vi "RSZVB Set PI Controller Mode.vi"(7 "PI Controller Mode (Auto)":i32(ring) items=["Auto", "Manual"], 8 "error in (no error)":errorcluster {"code" format="%.0x"}, 9 "Port (1)":i32=1, 10 "Channel (1)":i32=1, 11 "VISA session":refnum<visa-resource-name>) -> (0 "error out":errorcluster {"code" format="%.0x"}, 3 "dup VISA session":refnum<visa-resource-name>)   [LabVIEW 2011]
doc: "Enables automatic or manual setting of the PI controller parameters at source port <Pt>. \n\nRemote-control command(s):\nSOURce<Ch>:POWer<Pt>:ALC:PIParameter"
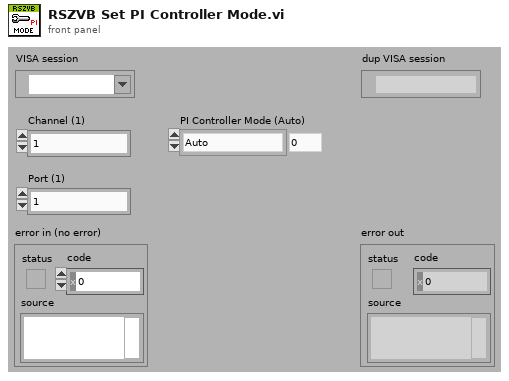
[diagram p1: front panel]
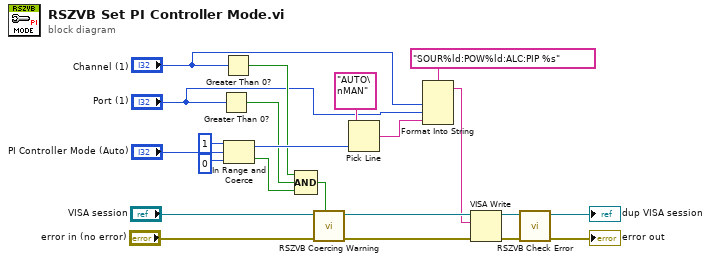
[diagram p0: block diagram]
diagram:
  n1 = Greater Than 0?(x="Port (1)") -> (x > 0?=w9:bool)
  n2 = Greater Than 0?(x="Channel (1)") -> (x > 0?=w10:bool)
  n3 = In Range and Coerce(upper limit=1, x="PI Controller Mode (Auto)", lower limit=0) -> (coerced(x)=w19:i32, In Range?=w8:bool)
  n4 = Compound Arithmetic op=AND(w10, w9, w8) -> (w7:bool)
  n5 = call "RSZVB Coercing Warning.vi"("In Range?"=w7, "error in (no error)"="error in (no error)", "VISA session"="VISA session") -> ("error out"=w16:errorcluster, "dup VISA session"=w17:refnum<visa-resource-name>)  [unwired: 7 in]
  n6 = Pick Line(multi-line string="AUTO\nMAN", line index=w19) -> (output string=w11:string)  [unwired: 1 in]
  n7 = Format Into String(format string="SOUR%ld:POW%ld:ALC:PIP %s", "Channel (1)", "Port (1)", w11) -> (resulting string=w13:string)  [unwired: 2 in, 1 out]
  n8 = VISA Write(VISA resource name=w17, write buffer=w13, error in (no error)=w16) -> (VISA resource name out=w14:refnum<visa-resource-name>, error out=w15:errorcluster)  [unwired: 1 out]
  n9 = call "RSZVB Check Error.vi"("error in (no error)"=w15, "VISA session"=w14) -> ("error out"=→"error out":errorcluster, "dup VISA session"=→"dup VISA session":refnum<visa-resource-name>)  [unwired: 8 in]
